vi "Set 1D Array String.vi"(5 "use temporary file? (F)":bool, 8 "error in":errorcluster, 9 "value":string[](array[string]), 10 "variable name":string, 11 "GOLPI ref. in":T1={"pipe handle"={"lv_proc.dll file path"=path "", "process instance handle"=[], "debug mode"=FALSE, "debug data"=[]}, "fast read timeout [ms]"=500, "fast read settle time [ms]"=10, "fast read to multiple [ms]"=1, "max elements per input line"=100, "slow read timeout [ms]"=5000, "stdin double format specifier"="%_16e", "max elements per stdout output column"=100, "console mode bitstream"=FALSE, "bitstream first read timeout [ms]"=1000, "bitstream read timeout [ms]"=50, "struct transfer possible"=FALSE, "matlab mode"=FALSE}) -> (0 "error out":errorcluster, 3 "GOLPI ref. out":T1={"pipe handle"={"lv_proc.dll file path"=path "", "process instance handle"=[], "debug mode"=FALSE, "debug data"=[]}, "fast read timeout [ms]"=500, "fast read settle time [ms]"=10, "fast read to multiple [ms]"=1, "max elements per input line"=100, "slow read timeout [ms]"=5000, "stdin double format specifier"="%_16e", "max elements per stdout output column"=100, "console mode bitstream"=FALSE, "bitstream first read timeout [ms]"=1000, "bitstream read timeout [ms]"=50, "struct transfer possible"=FALSE, "matlab mode"=FALSE})   [LabVIEW 2020, in "GOLPI library.lvlib"]
doc: "Part of polymorph Set Variable.vi"
uses:
  GOLPI library.lvlib
  GOLPI reference Type Def.ctl
  Pipe Handle.ctl
  LV Process library.lvlib
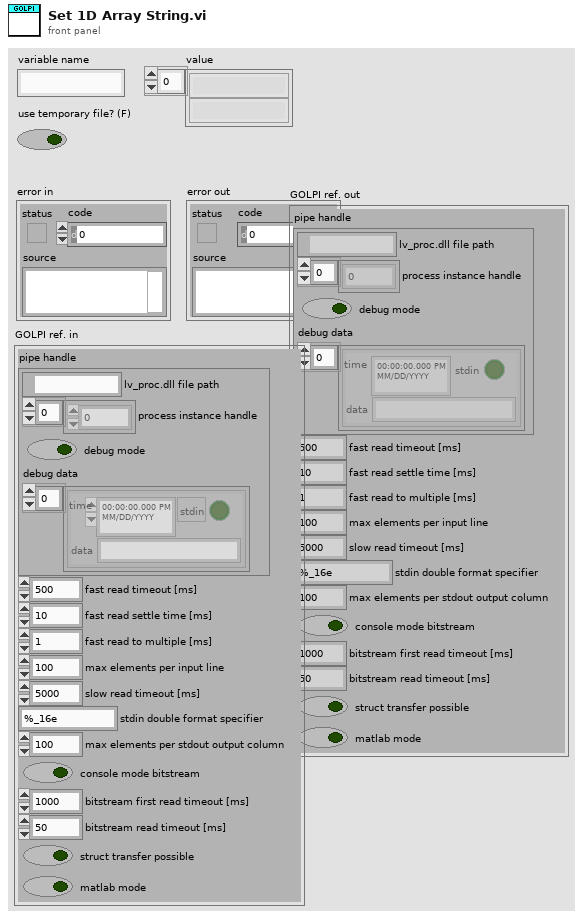
[diagram p1: front panel]
types:
  T1 = typedef "GOLPI library.lvlib/GOLPI reference Type Def.ctl" = cluster{"pipe handle":T2, "fast read timeout [ms]":u32, "fast read settle time [ms]":u32, "fast read to multiple [ms]":u32, "max elements per input line":u32, "slow read timeout [ms]":u32, "stdin double format specifier":string, "max elements per stdout output column":u32, "console mode bitstream":bool, "bitstream first read timeout [ms]":u32, "bitstream read timeout [ms]":u32, "struct transfer possible":bool, "matlab mode":bool}
  T2 = typedef "LV Process library.lvlib/Pipe Handle.ctl" = cluster{"lv_proc.dll file path":path, "process instance handle":u32[], "debug mode":bool, "debug data":cluster{"time":timestamp, "stdin":bool, "data":string}[]}
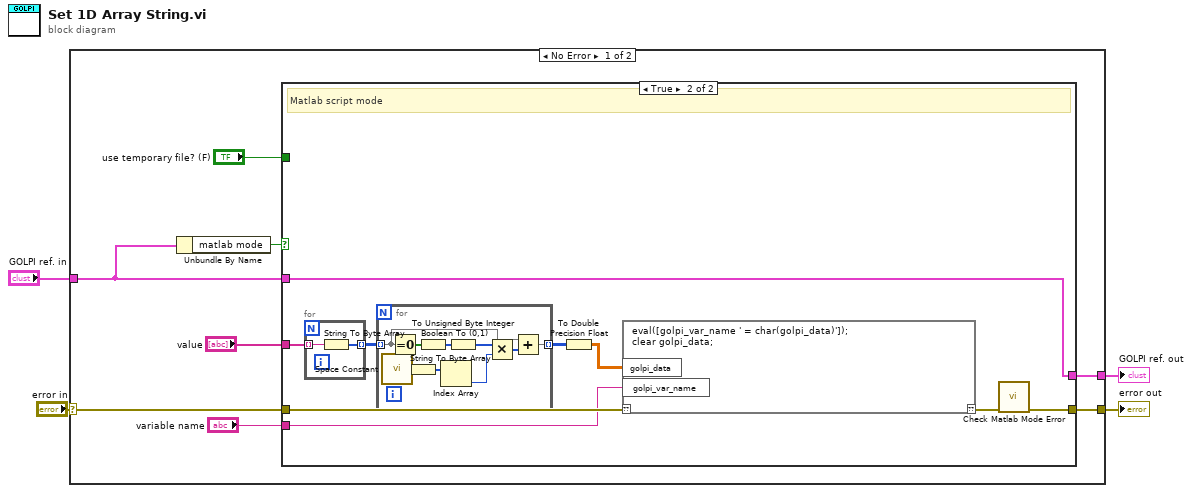
[diagram p0: block diagram]
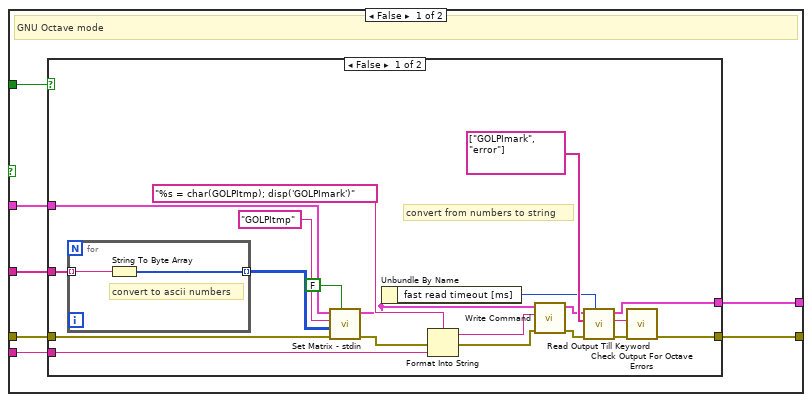
[diagram p2: hidden frame]
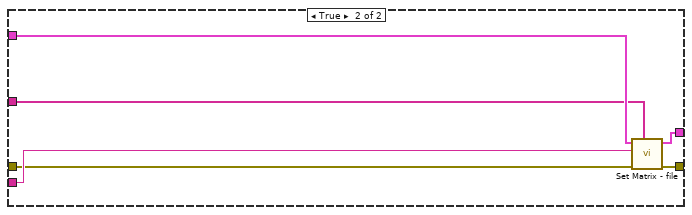
[diagram p3: hidden frame]
diagram:
  n1 = case shown="No Error" "error in" {
    selector: "error in" -> [w8 w69]
    tunnel: [w12 w69] -> w4
    tunnel: "GOLPI ref. in" -> [w6 w68]
    tunnel: [w11 w68] -> w1
    frame No Error {
      n2 = Unbundle By Name(w6) -> ("matlab mode"=w5:bool)
      n3 = case shown="True" w5 {
        tunnel: [w19 w48] -> w12
        tunnel: [w18 w50] -> w11
        tunnel: "variable name" -> [w17 w55]
        tunnel: "value" -> [w16 w54]
        tunnel: w8 -> [w15 w56]
        tunnel: w6 -> [w14 w50]
        tunnel: "use temporary file? (F)" -> [w13 _]
        frame False {
          # "GNU Octave mode"
          n4 = case shown="False" w13 {
            tunnel: [w39 w44] -> w19
            tunnel: [w38 w43] -> w18
            tunnel: w17 -> [w36 w47]
            tunnel: w16 -> [w22 w42]
            tunnel: w15 -> [w26 w45]
            tunnel: w14 -> [w25 w46]
            frame False {
              # "convert from numbers to string"
              n5 = for {
                tunnel: w22 -> [w41] mode=indexing
                tunnel: [w40] -> w21 mode=indexing
                # "convert to ascii numbers"
                n6 = String To Byte Array(string=w41) -> (unsigned byte array=w40:u8[])
              }
              n7 = call "Set Matrix - stdin.vi"("swap dimensions? (F)"=FALSE ("swap dimensions?"), "error in"=w26, "value"=w21, "variable name"="GOLPItmp", "GOLPI ref. in"=w25) -> ("error out"=w24:errorcluster, "GOLPI ref. out"=w23:T1)  [unwired: 5 in]
              n8 = Unbundle By Name(w23) -> ("fast read timeout [ms]"=w28:u32)
              n9 = Format Into String(format string="%s = char(GOLPItmp); disp('GOLPImark')", error in=w24, w36) -> (resulting string=w34:string, error out=w35:errorcluster)  [unwired: 1 in]
              n10 = call "Write Command.vi"("error in"=w35, "command"=w34, "GOLPI ref. in"=w23) -> ("error out"=w33:errorcluster, "GOLPI ref. out"=w30:T1)  [unwired: 7 in]
              n11 = call "Read Output Till Keyword.vi"("timeout [ms]"=w28, "error in"=w33, "keywords"=string[] ["GOLPImark", "error"], "GOLPI ref. in"=w30) -> ("error out"=w32:errorcluster, "read buffer"=w29:string, "GOLPI ref. out"=w38:T1)  [unwired: 4 in, 1 out]
              n12 = call "Check Output For Octave Errors.vi"("error in"=w32, "read buffer"=w29) -> ("error out"=w39:errorcluster)  [unwired: 9 in]
            }
            frame True {
              n13 = call "Set Matrix - file.vi"("string array"=w42, "error in (no error)"=w45, "variable name"=w47, "GOLPI ref. in"=w46) -> ("error out"=w44:errorcluster, "GOLPI ref. out"=w43:T1)  [unwired: 6 in]
            }
          }
        }
        frame True {
          # "Matlab script mode"
          n14 = for {
            tunnel: w54 -> [w67] mode=indexing
            tunnel: [w66] -> w53 mode=indexing
            n15 = String To Byte Array(string=w67) -> (unsigned byte array=w66:u8[])
          }
          n16 = for {
            tunnel: w53 -> [w58] mode=indexing
            tunnel: [w57] -> w52 mode=indexing
            n17 = call <vilib>:"Space Constant.vi"() -> ("String"=w63:string)
            n18 = Equal To 0?(x=w58) -> (x = 0?=w65:bool[])
            n19 = String To Byte Array(string=w63) -> (unsigned byte array=w62:u8[])
            n20 = Boolean To (0,1)(Boolean=w65) -> (0, 1=w64:i16[])
            n21 = Index Array(array=w62) -> (element=w61:u8)  [unwired: 1 in]
            n22 = To Unsigned Byte Integer(number=w64) -> (unsigned 8bit integer=w60:u8[])
            n23 = Multiply(x=w60, y=w61) -> (x*y=w59:u8[])
            n24 = Add(x=w58, y=w59) -> (x+y=w57:u8[])
          }
          n25 = To Double Precision Float(number=w52) -> (double precision float=w51:dbl[][])
          n26 = script code="eval([golpi_var_name ' = char(golpi_data)']);\nclear golpi_data;"("??"=w56, "golpi_var_name"=w55, "golpi_data"=w51) -> ("??"=w49:errorcluster)
          n27 = call "Check Matlab Mode Error.vi"("error in"=w49) -> ("error out"=w48:errorcluster)  [unwired: 10 in]
        }
      }
    }
    frame Error {
    }
  }
  "error out" <- w4
  "GOLPI ref. out" <- w1
